vi "initialize assembly lists.vi"(4 "output dictionary":refnum<class "data dictionary.lvclass">, 6 "input dictionary":refnum<class "data dictionary.lvclass">, 8 "error in":errorcluster, 10 "EthernetIP configuration in":refnum<class "EthernetIP configuration.lvclass">, 11 "EthernetIP runtime in":refnum<class "EthernetIP runtime.lvclass">) -> (0 "error out":errorcluster, 3 "EthernetIP runtime out":refnum<class "EthernetIP runtime.lvclass">)   [LabVIEW 2013, in "EthernetIP runtime.lvclass"]
uses:
  EthernetIP runtime.lvclass
  configuration/EthernetIP configuration.lvclass
  <vilib>/NI/Tag Bus/dictionary/data dictionary.lvclass
  <vilib>/ethernetip/ethernetip.llb/ethernetip.ctl
  assembly data spec.ctl
  conversion specification.ctl
  <vilib>/NI/Tag Bus/tag/Data Type.ctl
  configuration/EthernetIP configuration.lvclass/EthernetIP configuration.ctl
  <vilib>/ethernetip/ethernetip.llb/EthernetIPAssemblyType.ctl
  channel/EthernetIP Channel.lvclass/EthernetIP Channel.ctl
  <vilib>/NI/Tag Bus/tag/tag descriptor.lvclass/tag descriptor.ctl
  <vilib>/NI/Tag Bus Module Framework/channel/TBM channel.lvclass/TBM channel.ctl
  EthernetIP runtime.lvclass/EthernetIP runtime.ctl
  channel/Read Instance ID.vi
  <vilib>/NI/Tag Bus/tag/read tag name.vi
  <vilib>/NI/Tag Bus Module Framework/channel/Read channel classification.vi
  <vilib>/NI/Tag Bus/tag/read data type.vi
  channel/Read byte index.vi
  channel/Read subindex.vi
  configuration/Read assemblies.vi
  configuration/read eip channels.vi
  channel/EthernetIP Channel.lvclass
  <vilib>/NI/Tag Bus/tag/tag descriptor.lvclass
  <vilib>/ethernetip/ethernetip.lvlib
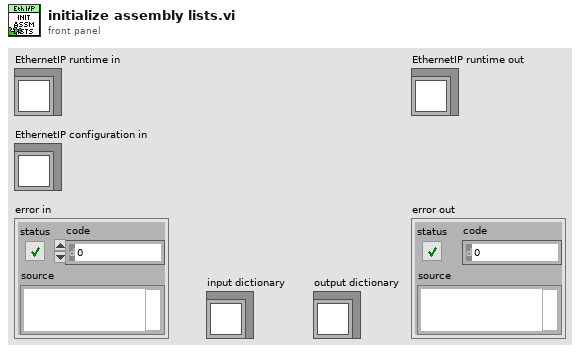
[diagram p1: front panel]
types:
  T1 = typedef "EthernetIP runtime.lvclass/assembly data spec.ctl" = cluster{"Instance ID":u32, "specification":T2[]}
  T2 = typedef "EthernetIP runtime.lvclass/conversion specification.ctl" = cluster{"data type":T3, "data index":i32, "byte index":i32, "subindex":i32}
  T3 = typedef "tag bus.lvlib/tag descriptor.lvclass/Data Type.ctl" = enum16{"Double", "Single", "I64", "I32", "I16", "I8", "U64", "U32", "U16", "U8", "Boolean", "String", "Array of Double", "Array of Single", "Array of I64", "Array of I32", "Array of I16", "Array of I8", "Array of U64", "Array of U32", "Array of U16", "Array of U8", "Array of Boolean", "Array of String"}
  T4 = typedef "ethernetip.lvlib/ethernetip.ctl" = refnum<k21>
  T5 = typedef "EthernetIP configuration.lvclass/assembly definition.ctl" = cluster{"name":string, "Instance ID":u32, "Type":T6, "Size (bytes)":u32}
  T6 = typedef "EthernetIP configuration.lvclass/assembly type.ctl" = enum32{"Producing", "Consuming"}
  T7 = typedef "ethernetip.lvlib/EthernetIPAssemblyType.ctl" = enum16{"Producing", "Consuming", "Configuration"}
  T8 = typedef "TBM channel.lvclass/channel classification.ctl" = enum16{"input data", "output data", "processing parameter", "processing result"}
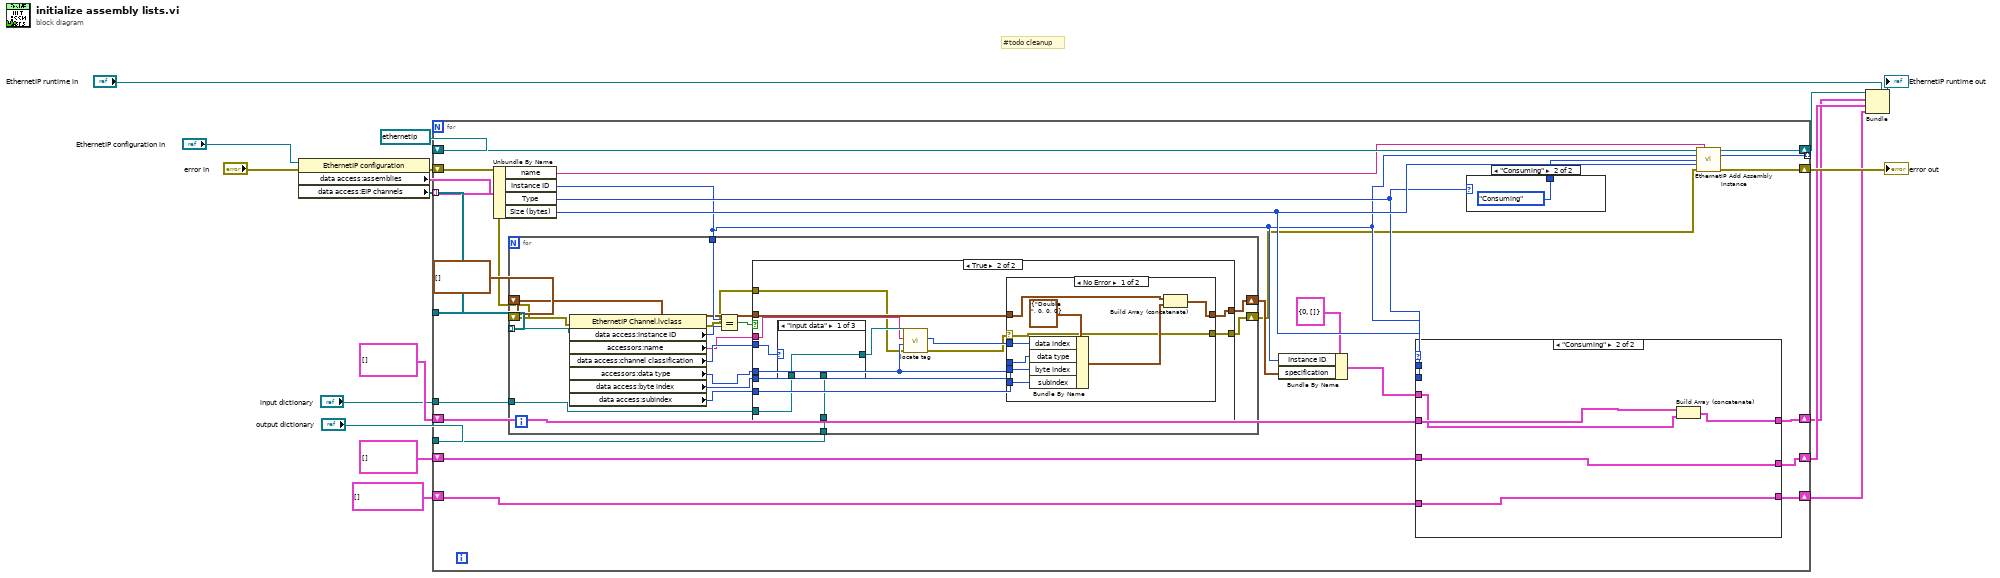
[diagram p0: block diagram]
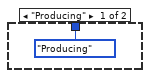
[diagram p6: hidden frame]
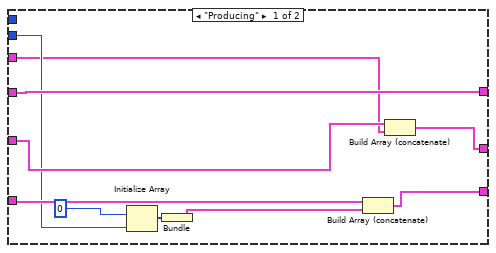
[diagram p7: hidden frame]
diagram:
  # "#todo cleanup"
  n1 = property class="EthernetIP configuration"(reference="EthernetIP configuration in", error in="error in") -> (error out=w14:errorcluster, "data access:assemblies"=w17:T5[], "data access:EIP channels"=w18:refnum<class "EthernetIP Channel.lvclass">[])  [unwired: 1 out]
  n2 = for {
    shift-right: [w43] -> w11
    shift-left: w14 -> [w22]
    shift-right: [w42] -> w13
    shift-left: T4 "Default" ("Session in") -> [w41]
    tunnel: w17 -> [w40] mode=indexing
    tunnel: [w38] -> _ mode=indexing
    tunnel: w18 -> [w28]
    shift-right: [w29] -> w3
    shift-left: T1[] [] ("output assemblies") -> [w30]
    shift-right: [w34] -> w4
    shift-left: T1[] [] ("output assemblies") -> [w33]
    shift-right: [w31] -> w5
    shift-left: cluster{"output allocation":u8[]}[] [] ("output allocations") -> [w32]
    tunnel: "input dictionary" -> [w20]
    tunnel: "output dictionary" -> [w19]
    n3 = Unbundle By Name(w40) -> ("name"=w39:string, "Instance ID"=w25:u32, "Type"=w36:T6, "Size (bytes)"=w37:u32)
    n4 = for {
      tunnel: w28 -> [w59] mode=indexing
      tunnel: w25 -> [w58]
      shift-right: [w57] -> w24
      shift-left: T2[] [] ("specification") -> [w56]
      shift-right: [w44] -> w21
      shift-left: w22 -> [w50]
      tunnel: w20 -> [w48]
      tunnel: w19 -> [w47]
      n5 = property class="EthernetIP Channel.lvclass"(reference=w59, error in=w50) -> (error out=w45:errorcluster, "data access:Instance ID"=w51:u32, "accessors:name"=w46:string, "data access:channel classification"=w49:T8, "accessors:data type"=w52:T3, "data access:byte index"=w53:i32, "data access:subindex"=w54:i32)  [unwired: 1 out]
      n6 = Equal?(x=w58, y=w51) -> (x = y?=w55:bool)
      n7 = case shown="True" w55 {
        tunnel: [w61 w75] -> w57
        tunnel: w56 -> [w61 w74]
        tunnel: w54 -> [_ w73]
        tunnel: w53 -> [_ w72]
        tunnel: w52 -> [_ w66]
        tunnel: w49 -> [_ w71]
        tunnel: w48 -> [_ w70]
        tunnel: w47 -> [_ w69]
        tunnel: w46 -> [_ w67]
        tunnel: w45 -> [w60 w65]
        tunnel: [w60 w62] -> w44
        frame False {
        }
        frame True {
          n8 = case shown="\"input data\"" w71 {
            tunnel: w70 -> [w76 _ _]
            tunnel: w69 -> [_ _ w77]
            tunnel: [w76 _ w77] -> w68
            frame "input data" {
            }
            frame Default {
            }
            frame "output data" {
            }
          }
          n9 = call <vilib>:"locate tag.vi"("error in"=w65, "data type"=w66, "name"=w67, "data dictionary in"=w68) -> ("error out"=w63:errorcluster, "index"=w64:i32)  [unwired: 5 in, 1 out]
          n10 = case shown="No Error" w63 {
            selector: w63 -> [w78 w87]
            tunnel: [w80 w88] -> w75
            tunnel: w74 -> [w81 w88]
            tunnel: w73 -> [w85 _]
            tunnel: w72 -> [w84 _]
            tunnel: w66 -> [w83 _]
            tunnel: w64 -> [w79 _]
            tunnel: [w78 w87] -> w62
            frame No Error {
              n11 = Bundle By Name(cluster=T2 {"data type"=enum."Double", "data index"=0, "byte index"=0, "subindex"=0} ("specification"), "data index"=w79, "data type"=w83, "byte index"=w84, "subindex"=w85) -> (w82:T2)
              n12 = Build Array (concatenate)(w81, w82) -> (w80:T2[])
            }
            frame Error {
            }
          }
        }
      }
    }
    n13 = Bundle By Name(cluster=T1 {"Instance ID"=0, "specification"=[]} ("assembly data spec"), "Instance ID"=w25, "specification"=w24) -> (w23:T1)
    n14 = case shown="\"Consuming\"" w36 {
      tunnel: w25 -> [_ _]
      tunnel: w37 -> [w95 _]
      tunnel: [w100 w105] -> w34
      tunnel: w33 -> [w99 w105]
      tunnel: w32 -> [w97 w104]
      tunnel: [w98 w104] -> w31
      tunnel: w30 -> [w96 w103]
      tunnel: [w96 w102] -> w29
      tunnel: w23 -> [w91 w101]
      frame "Producing" {
        n15 = Initialize Array(u8 0, w95) -> (w93:u8[])
        n16 = Bundle(w93) -> (w92:cluster{u8[]})  [unwired: 1 in]
        n17 = Build Array (concatenate)(w97, w92) -> (w98:cluster{"output allocation":u8[]}[])
        n18 = Build Array (concatenate)(w99, w91) -> (w100:T1[])
      }
      frame "Consuming" {
        n19 = Build Array (concatenate)(w103, w101) -> (w102:T1[])
      }
    }
    n20 = case shown="\"Consuming\"" w36 {
      tunnel: [EthernetIPAssemblyType."Producing" ("Type") EthernetIPAssemblyType."Consuming" ("Type")] -> w35
      frame "Producing" {
      }
      frame "Consuming" {
      }
    }
    n21 = call <vilib>:"EthernetIP Add Assembly Instance.vi"("Session in"=w41, "Name (optional)"=w39, "Instance ID in"=w25, "Type"=w35, "Size (bytes)"=w37, "error in"=w21) -> ("Session out"=w42:T4, "Instance ID out"=w38:u32, "error out"=w43:errorcluster)  [unwired: 7 in]
  }
  "error out" <- w11
  n22 = Bundle(cluster="EthernetIP runtime in", w13, w3, w4, w5) -> (→"EthernetIP runtime out":refnum<class "EthernetIP runtime.lvclass">)
